vi "daqmx_trigger internally_test.vi"   [LabVIEW 2013]
uses:
  <vilib>/DAQmx/write.llb/DAQmx Write.vi
  <vilib>/DAQmx/write.llb/DAQmx Write (Analog 1D Wfm NChan NSamp).vi
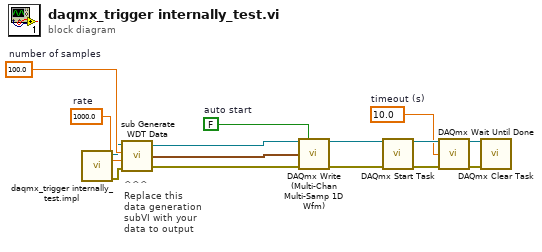
[diagram p0: block diagram]
diagram:
  w6 = 10.0  # timeout (s)
  w10 = 1000.0  # rate
  w11 = 100.0  # number of samples
  w15 = FALSE  # auto start
  # "^^^\nReplace this\ndata generation\nsubVI with your\ndata to output"
  n1 = call "daqmx_trigger internally_test.impl.vi"() -> ("error out"=w1:errorcluster, "task out"=w2:refnum<k21>)  [unwired: 10 in]
  n2 = call <vilib>:"sub Generate WDT Data.vi"("task in"=w2, "number of samples"=w11, "update rate"=w10, "error in"=w1) -> ("task out"=w13:refnum<k21>, "Data"=w12:waveform(dbl)[], "error out"=w14:errorcluster)  [unwired: 1 in]
  n3 = call-poly "DAQmx Write (Multi-Chan Multi-Samp 1D Wfm).vi"("task/channels in"=w13, "auto start"=w15, "data"=w12, "error in"=w14) -> ("task out"=w5:refnum<k21>, "error out"=w4:errorcluster)  [unwired: 9 in, 1 out]
  n4 = call <vilib>:"DAQmx Start Task.vi"("task/channels in"=w5, "error in"=w4) -> ("task out"=w9:refnum<k21>, "error out"=w8:errorcluster)  [unwired: 12 in]
  n5 = call <vilib>:"DAQmx Wait Until Done.vi"("task/channels in"=w9, "timeout (sec)"=w6, "error in"=w8) -> ("task out"=w3:refnum<k21>, "error out"=w7:errorcluster)  [unwired: 11 in]
  n6 = call <vilib>:"DAQmx Clear Task.vi"("task in"=w3, "error in"=w7) -> ()  [unwired: 13 in, 1 out]
